vi "Edit-dialog.vi"(8 "error in (no error)":errorcluster, 11 "Action in":refnum<class "Substrate.lvclass">) -> (0 "error out":errorcluster, 3 "Action out":refnum<class "Substrate.lvclass">)   [LabVIEW 2013, in "PowderDeposition.lvlib" / "Substrate.lvclass"]
uses:
  Substrate.lvclass
  Move-Absolute/Move-Absolute-settings.ctl
  Substrate.lvclass/Substrate.ctl
  Move-Absolute/Move-Absolute.lvclass
panel:
  in  "Cancel":bool
  in  "OK":bool
  in  "Edit dialog":T1
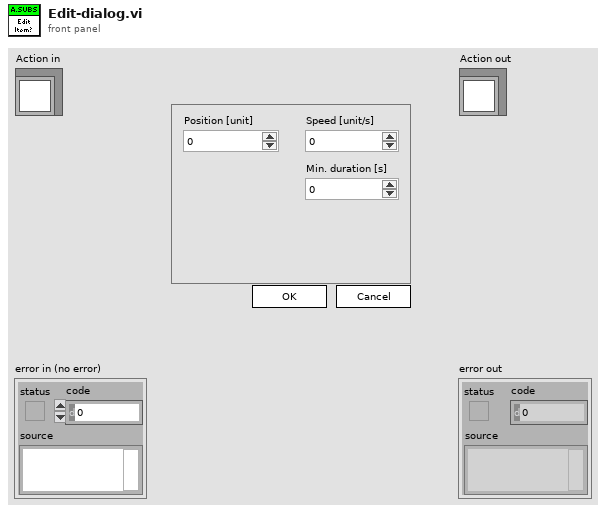
[diagram p1: front panel]
types:
  T1 = typedef "PowderDeposition.lvlib/Move-Absolute.lvclass/Move-Absolute-settings.ctl" = cluster{"Position":dbl, "Speed":dbl, "Min duration":dbl}
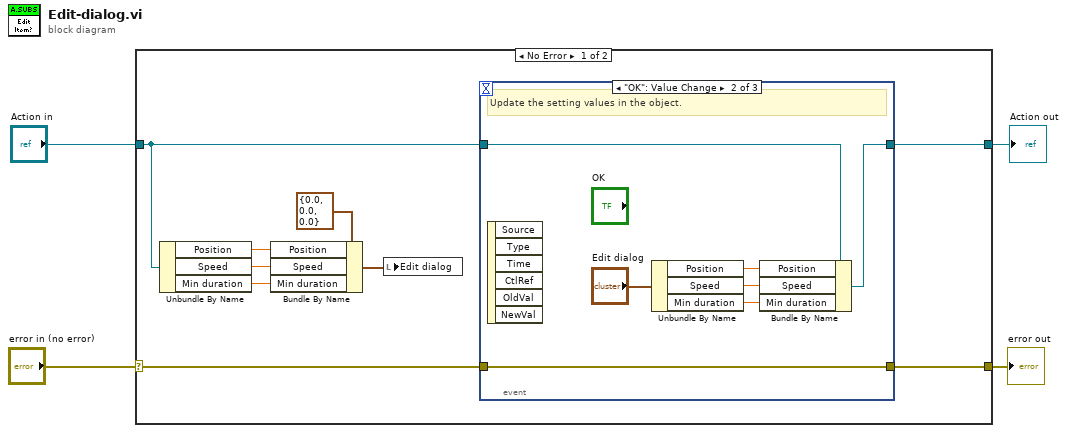
[diagram p0: block diagram]
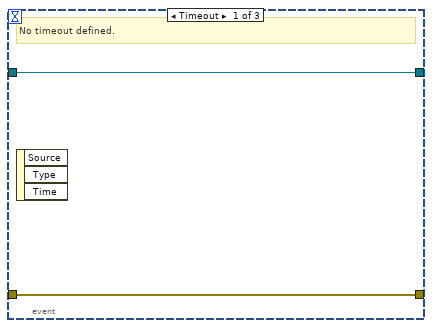
[diagram p2: hidden frame]
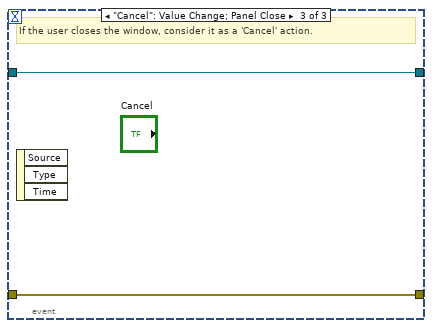
[diagram p3: hidden frame]
diagram:
  n1 = case shown="No Error" "error in (no error)" {
    selector: "error in (no error)" -> [w12 w26]
    tunnel: [w11 w26] -> w3
    tunnel: [w13 w25] -> w1
    tunnel: "Action in" -> [w5 w25]
    frame No Error {
      n2 = Unbundle By Name(w5) -> ("Position"=w8:dbl, "Speed"=w9:dbl, "Min duration"=w10:dbl)
      n3 = Bundle By Name(cluster=T1 {"Position"=0.0, "Speed"=0.0, "Min duration"=0.0} ("Edit dialog"), "Position"=w8, "Speed"=w9, "Min duration"=w10) -> (w6:T1)
      n4 = local write "Edit dialog"(w6) -> ()
      n5 = event shown="[1] \"OK\": Value Change" {
        selector: _ -> [_ _ _]
        dyn-events: _ -> [_ _ _]
        timeout: _ -> [_ _ _]
        tunnel: w5 -> [w15 w21 w24]
        tunnel: [w15 w20 w24] -> w13
        tunnel: w12 -> [w14 w22 w23]
        tunnel: [w14 w22 w23] -> w11
        event Timeout {
          # "No timeout defined."
          n6 = event-data() -> ()  [unwired: 1 in, 3 out]
        }
        event "OK": Value Change {
          # "Update the setting values in the object."
          n7 = event-data() -> ()  [unwired: 1 in, 6 out]
          n8 = Unbundle By Name("Edit dialog") -> ("Position"=w17:dbl, "Speed"=w18:dbl, "Min duration"=w16:dbl)
          n9 = Bundle By Name(cluster=w21, "Position"=w17, "Speed"=w18, "Min duration"=w16) -> (w20:refnum<class "Substrate.lvclass">)
        }
        event "Cancel": Value Change; Panel Close {
          # "If the user closes the window, consider it as a 'Cancel' action."
          n10 = event-data() -> ()  [unwired: 1 in, 3 out]
        }
      }
    }
    frame Error {
    }
  }
  "error out" <- w3
  "Action out" <- w1
